vi "ep_Get Peak in Window.vi"(8 "error in (no error)":errorcluster, 9 "sinc interpolation? (F)":bool, 10 "sideband window":T1={"sideband frequency"=0.0, "number of half window length "=1, "fbrb in range? (F)"=FALSE}, 11 "spectra points":T2) -> (0 "error out":errorcluster, 1 "output valid? (F)":bool, 2 "magnitude [dB]":dbl, 3 "frequency":dbl)   [LabVIEW 2014, in "NI_EP_Motor Monitoring.lvlib"]
uses:
  <vilib>/addons/Electrical Power/Motor Monitoring/NI_EP_Motor Monitoring.lvlib
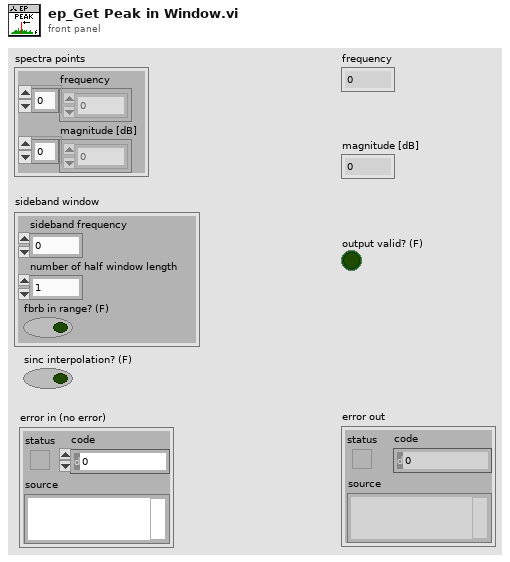
[diagram p1: front panel]
types:
  T1 = cluster{"sideband frequency":dbl, "number of half window length ":u8, "fbrb in range? (F)":bool}
  T2 = cluster{"frequency":dbl[], "magnitude [dB]":dbl[]}
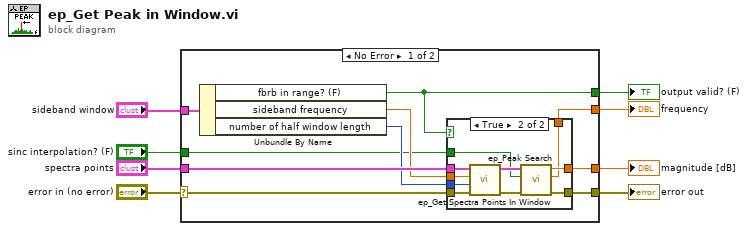
[diagram p0: block diagram]
diagram:
  n1 = case shown="No Error" "error in (no error)" {
    selector: "error in (no error)" -> [w17 w30]
    tunnel: "spectra points" -> [w18 _]
    tunnel: [w14 _] -> w4
    tunnel: [w16 w30] -> w6
    tunnel: "sideband window" -> [w15 _]
    tunnel: [w12 _] -> w3
    tunnel: [w10 _] -> w2
    tunnel: "sinc interpolation? (F)" -> [w9 _]
    frame No Error {
      n2 = Unbundle By Name(w15) -> ("fbrb in range? (F)"=w12:bool, "sideband frequency"=w11:dbl, "number of half window length"=w13:u8)
      n3 = case shown="True" w12 {
        tunnel: w18 -> [_ w29]
        tunnel: w17 -> [w19 w27]
        tunnel: [w19 w25] -> w16
        tunnel: [_ w24] -> w14
        tunnel: w11 -> [_ w23]
        tunnel: w13 -> [_ w22]
        tunnel: [_ w21] -> w10
        tunnel: w9 -> [_ w20]
        frame False {
        }
        frame True {
          n4 = call <vilib>:"ep_Get Spectra Points In Window.vi"("error in (no error)"=w27, "points of half window length"=w22, "sideband center frequency"=w23, "all spectra points"=w29) -> ("error out"=w26:errorcluster, "spectra points in window"=w28:cluster{"frequency":dbl[], "magnitude":dbl[]})  [unwired: 6 in]
          n5 = call <vilib>:"ep_Peak Search.vi"("error in (no error)"=w26, "sinc interpolation? (F)"=w20, "spectra points in window"=w28) -> ("error out"=w25:errorcluster, "interpolated peak frequency"=w21:dbl, "interpolated peak magnitude [dB]"=w24:dbl)  [unwired: 6 in]
        }
      }
    }
    frame Error {
    }
  }
  "error out" <- w6
  "frequency" <- w2
  "magnitude [dB]" <- w4
  "output valid? (F)" <- w3
